vi "KE2260B Read Circuit Breaker Status.vi"(8 "error in (no error)":errorcluster, 11 "VISA resource name":refnum<visa-resource-name>) -> (0 "error out":errorcluster, 2 "Circuit Breaker?":bool, 3 "VISA resource name out":refnum<visa-resource-name>)   [LabVIEW 2009, in "Keithley 2260B.lvlib"]
doc: "Queries the power switch trip setting (circuit breaker) of the power supply."
uses:
  <instrlib>/Keithley 2260B/Keithley 2260B.lvlib
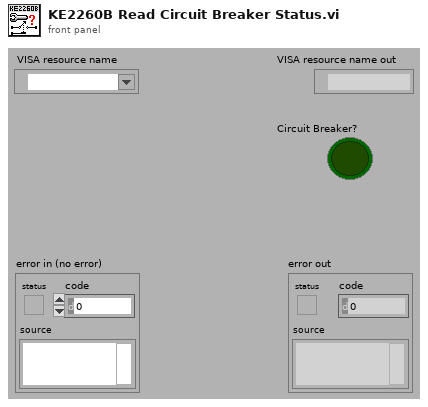
[diagram p1: front panel]
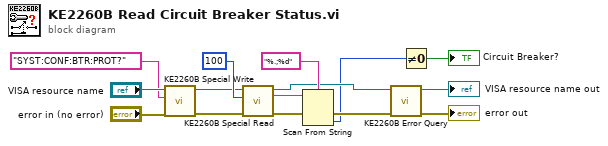
[diagram p0: block diagram]
diagram:
  n1 = call <instrlib>:"KE2260B Special Write.vi"("error in (no error)"="error in (no error)", "Write Buffer (\"\")"="SYST:CONF:BTR:PROT?" ("write buffer"), "VISA session"="VISA resource name") -> ("error out"=w6:errorcluster, "dup VISA session"=w2:refnum<visa-resource-name>)  [unwired: 6 in, 1 out]
  n2 = call <instrlib>:"KE2260B Special Read.vi"("error in (no error)"=w6, "byte count"=u32 100, "VISA session"=w2) -> ("error out"=w10:errorcluster, "read buffer"=w12:string, "dup VISA session"=w8:refnum<visa-resource-name>)  [unwired: 5 in, 1 out]
  n3 = Scan From String(format string="%.;%d", input string=w12, error in=w10) -> (error out=w9:errorcluster, output 1=w1:i32)  [unwired: 2 in, 2 out]
  n4 = call <instrlib>:"KE2260B Error Query.vi"("error in (no error)"=w9, "VISA resource name"=w8) -> ("error out"=→"error out":errorcluster, "VISA resource name out"=→"VISA resource name out":refnum<visa-resource-name>)  [unwired: 6 in, 2 out]
  n5 = Not Equal To 0?(x=w1) -> (x != 0?=→"Circuit Breaker?":bool)
